vi "DrawShots_save.vi"(1 "MainCluster_IN":T11) -> (0 "MainCluster_OUT":T11)   [LabVIEW 2019]
uses:
  move_dir_ud.ctl
  73093f7f-2ca4-43a7-b6b0-9389dd3223a1.vi
  move_dir_lr.ctl
  InvaderPositionArray.ctl
  <vilib>/picture/picture.llb/imagedata.ctl
  ShotInitCluster.ctl
  CharacterCluster.ctl
  <vilib>/Utility/miscctls.llb/LVPositionTypeDef.ctl
  <vilib>/Utility/miscctls.llb/LVBoundsTypeDef.ctl
  ShotCluster.ctl
  InitCluster.ctl
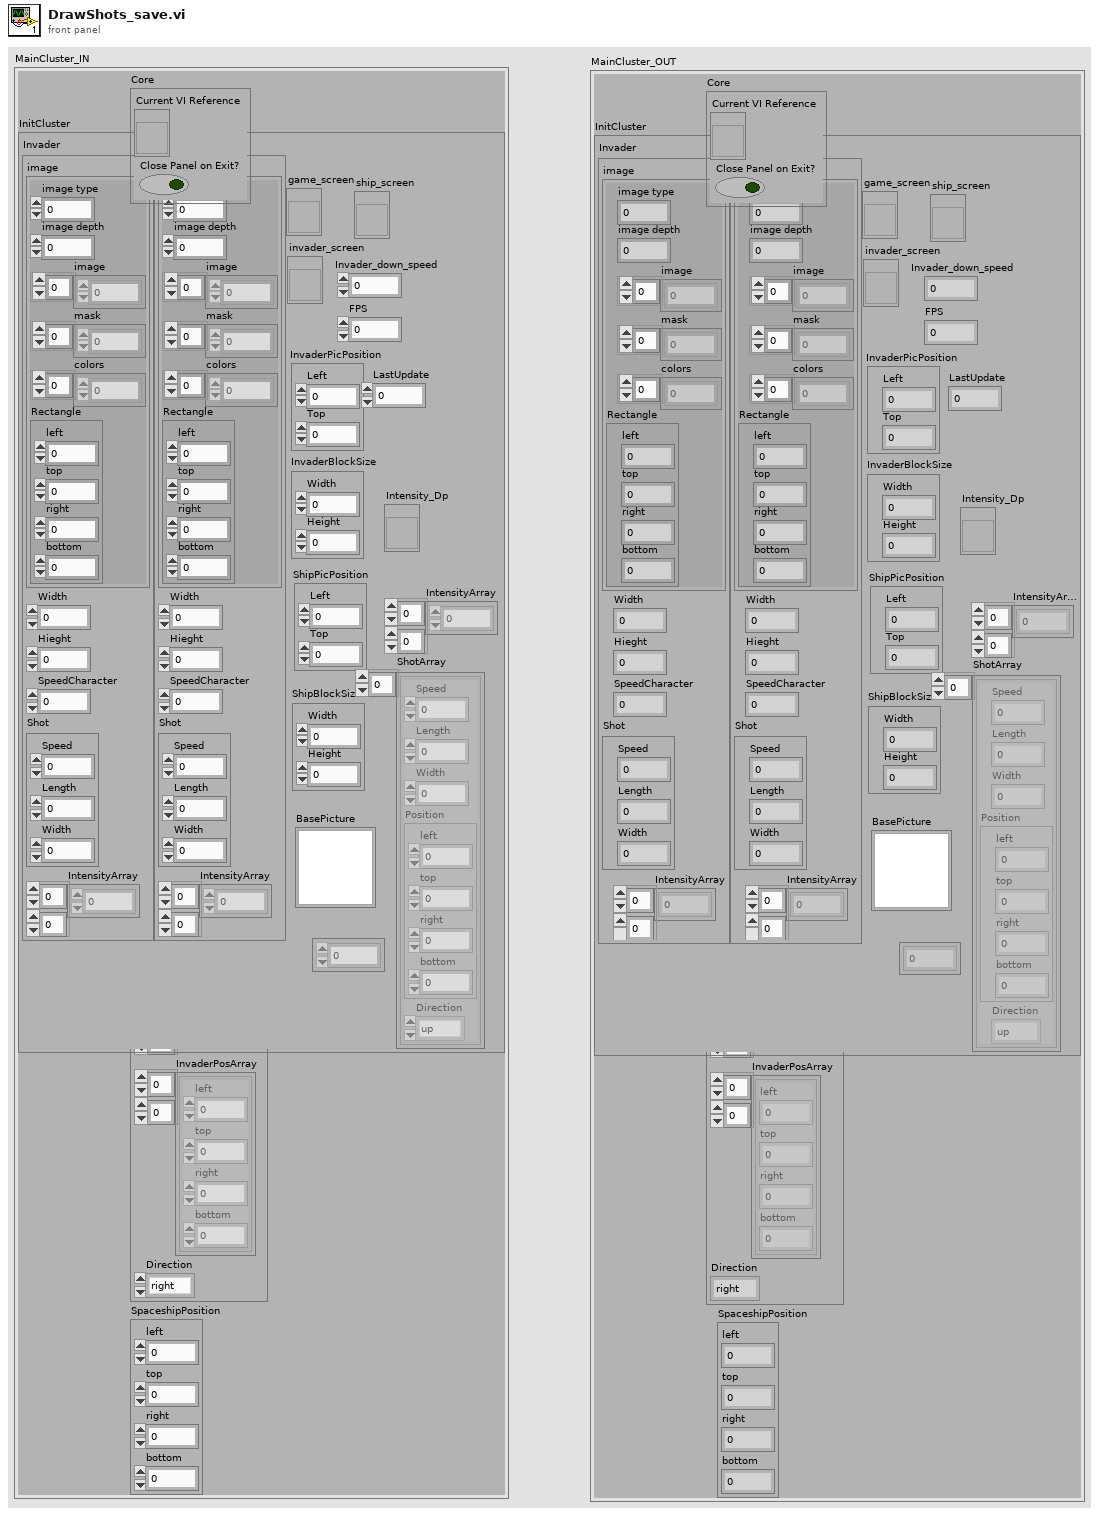
[diagram p1: front panel]
types:
  T1 = typedef "InitCluster.ctl" = cluster{"Invader":T2, "Spaceship":T2, "game_screen":refnum<vi>, "BasePicture":picture, "invader_screen":refnum<vi>, "InvaderPicPosition":T5, "Invader_down_speed":i16, "FPS":u16, "InvaderBlockSize":T6, "ship_screen":refnum<vi>, "ShipBlockSize":T6, "ShipPicPosition":T5, "LastUpdate":u32, "Intensity_Dp":refnum<vi>, "IntensityArray":u8[][], "ShotArray":T7[], "InvaderShotTimeArray":u32[]}
  T2 = typedef "CharacterCluster.ctl" = cluster{"image":T3, "Width":u32, "Hieght":u32, "SpeedCharacter":u32, "Shot":T4, "IntensityArray":u8[][]}
  T3 = typedef "imagedata.ctl" = cluster{"image type":i32, "image depth":i32, "image":u8[], "mask":u8[], "colors":u32[], "Rectangle":cluster{"left":i16, "top":i16, "right":i16, "bottom":i16}}
  T4 = typedef "ShotInitCluster.ctl" = cluster{"Speed":u32, "Length":u32, "Width":u32}
  T5 = typedef "LVPositionTypeDef.ctl" = cluster{"Left":i32, "Top":i32}
  T6 = typedef "LVBoundsTypeDef.ctl" = cluster{"Width":u32, "Height":u32}
  T7 = typedef "ShotCluster.ctl" = cluster{"Speed":u32, "Length":u32, "Width":u32, "Position":cluster{"left":i16, "top":i16, "right":i16, "bottom":i16}, "Direction":T8}
  T8 = typedef "move_dir_ud.ctl" = enum16{"up", "down"}
  T9 = typedef "InvaderPositionArray.ctl" = cluster{"InvaderAlive":bool[][], "InvaderPosArray":cluster{"left":i16, "top":i16, "right":i16, "bottom":i16}[][], "Direction":T10}
  T10 = typedef "move_dir_lr.ctl" = enum16{"right", "left"}
  T11 = cluster{"Core":cluster{"Current VI Reference":refnum<vi>, "Close Panel on Exit?":bool}, "InitCluster":T1, "InvaderPosArray":T9, "SpaceshipPosition":cluster{"left":i16, "top":i16, "right":i16, "bottom":i16}}
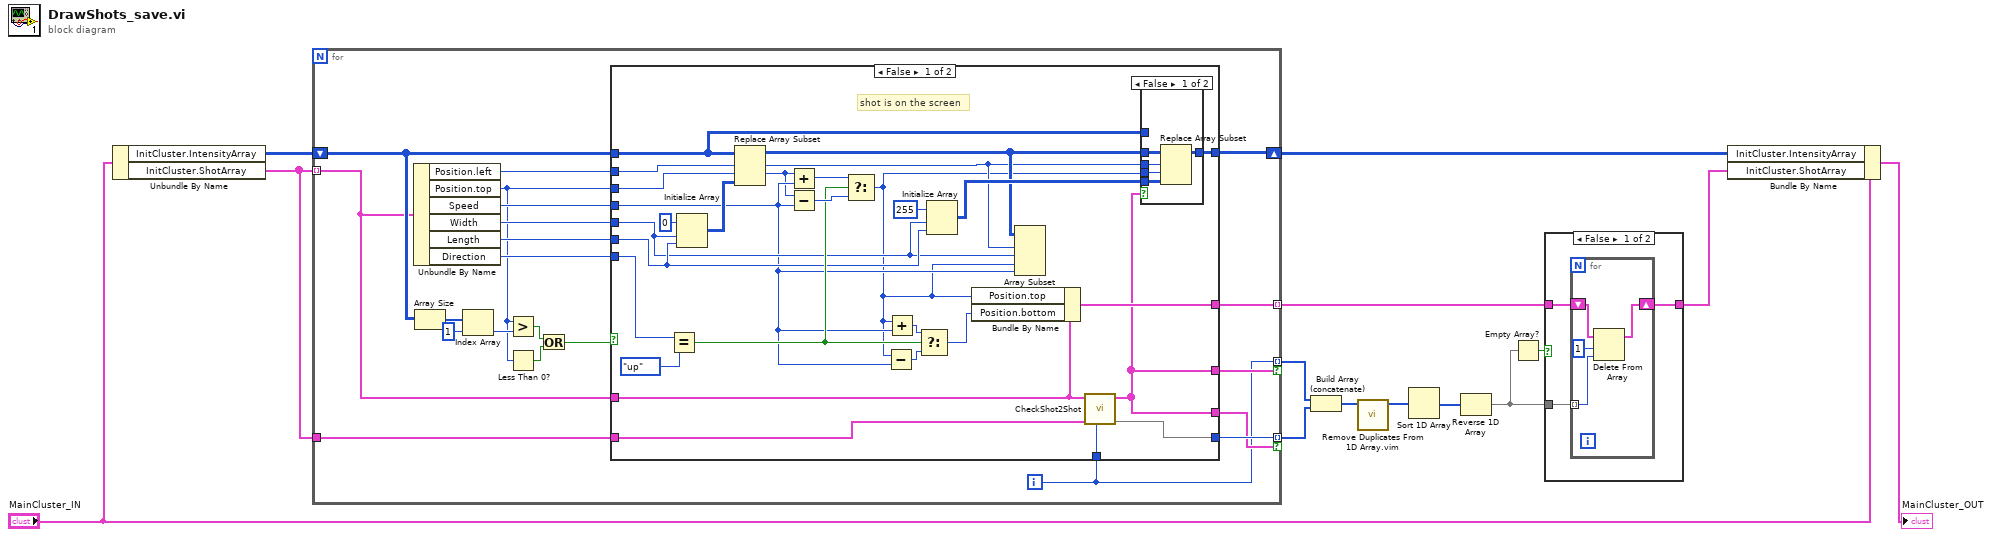
[diagram p0: block diagram]
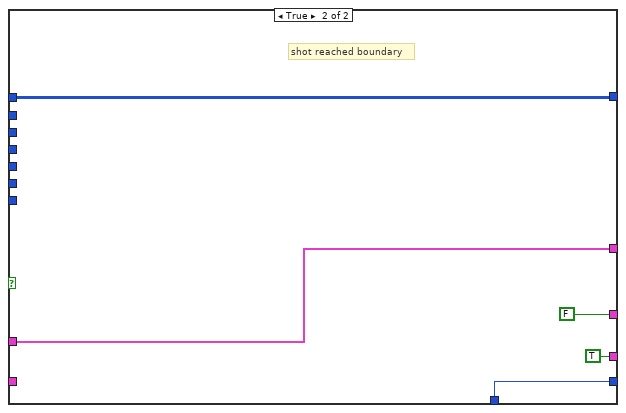
[diagram p4: hidden frame]
diagram:
  n1 = Unbundle By Name("MainCluster_IN") -> ("InitCluster.IntensityArray"=w14:u8[][], "InitCluster.ShotArray"=w10:T7[])
  n2 = for {
    tunnel: w10 -> [w18] mode=indexing
    shift-right: [w35] -> w13
    shift-left: w14 -> [w28]
    tunnel: [w33] -> w5 mode=indexing
    tunnel: w10 -> [w19]
    tunnel: [w15] -> w9 mode=indexing if=w20
    tunnel: [w17] -> w8 mode=indexing if=w16
    i -> [w15]
    n3 = Unbundle By Name(w18) -> ("Position.left"=w29:i16, "Position.top"=w24:i16, "Speed"=w30:u32, "Width"=w31:u32, "Length"=w32:u32, "Direction"=w34:T8)
    n4 = Array Size(array=w28) -> (size(s)=w27:i32[])
    n5 = Index Array(array=w27, index=1) -> (element=w25:i32)
    n6 = Greater?(x=w24, y=w25) -> (0:w23:bool)
    n7 = Less Than 0?(x=w24) -> (x < 0?=w22:bool)
    n8 = Or(x=w23, y=w22) -> (x .or. y?=w21:bool)
    n9 = case shown="False" w21 {
      tunnel: [w60 w73] -> w35
      tunnel: w34 -> [w57 _]
      tunnel: w18 -> [w37 w72]
      tunnel: [w39 w72] -> w33
      tunnel: [w38 FALSE] -> w20
      tunnel: w32 -> [w48 _]
      tunnel: w31 -> [w47 _]
      tunnel: w30 -> [w46 _]
      tunnel: w29 -> [w45 _]
      tunnel: w28 -> [w43 w73]
      tunnel: w24 -> [w44 _]
      tunnel: w19 -> [w42 _]
      tunnel: [w41 w70] -> w17
      tunnel: [w38 TRUE ("Collision")] -> w16
      tunnel: w15 -> [w40 w70]
      frame False {
        # "shot is on the screen"
        n10 = Equal?(x=w57, y=move_dir_ud."up" ("Direction")) -> (x = y?=w53:bool)
        n11 = Initialize Array(u32 0 ("element"), w47, w48) -> (w61:u32[][])
        n12 = Replace Array Subset(array=w43, new element=w61, index (row)=w45, index (col)=w44) -> (w50:u8[][])
        n13 = Add(x=w44, y=w46) -> (x+y=w55:u32)
        n14 = Subtract(x=w44, y=w46) -> (x-y=w54:u32)
        n15 = Select(t=w55, s=w53, f=w54) -> (s? t:f=w36:u32)
        n16 = Subtract(x=w36, y=w46) -> (x-y=w51:u32)
        n17 = Add(x=w36, y=w46) -> (x+y=w52:u32)
        n18 = Select(t=w52, s=w53, f=w51) -> (s? t:f=w49:u32)
        n19 = Initialize Array(u32 255 ("element"), w47, w48) -> (w58:u32[][])
        n20 = Bundle By Name(cluster=w37, "Position.top"=w36, "Position.bottom"=w49) -> (w39:T7)
        n21 = Array Subset(array=w50, index (row)=w45, length (row)=w47, index (col)=w36, length (col)=w46) -> ()  [unwired: 1 out]
        n22 = call "CheckShot2Shot.vi"(6:w40, 8:w42, "ShotArray_IN"=w37) -> (0:w41, "ShotArray_OUT"=w38:T7[])  [unwired: 7 in]
        n23 = case shown="False" w38 {
          tunnel: [w67 w68] -> w60
          tunnel: w58 -> [w66 _]
          tunnel: w50 -> [w65 w68]
          tunnel: w45 -> [w64 _]
          tunnel: w36 -> [w63 _]
          tunnel: w43 -> [_ _]
          frame False {
            n24 = Replace Array Subset(array=w65, new element=w66, index (row)=w64, index (col)=w63) -> (w67:u8[][])
          }
          frame True {
          }
        }
      }
      frame True {
        # "shot reached boundary"
      }
    }
  }
  n25 = Build Array (concatenate)(w9, w8) -> (w3:i32[])
  n26 = call "Remove Duplicates From 1D Array.vim"("array"=w3) -> ("array with duplicates removed"=w7:i32[])  [unwired: 10 in]
  n27 = Sort 1D Array(array=w7) -> (sorted array=w6:i32[])
  n28 = Reverse 1D Array(array=w6) -> (reversed array=w2:i32[])
  n29 = Empty Array?(array=w2) -> (empty?=w1:bool)
  n30 = case shown="False" w1 {
    tunnel: w2 -> [w76 _]
    tunnel: w5 -> [w75 w81]
    tunnel: [w74 w81] -> w4
    frame False {
      n31 = for {
        tunnel: w76 -> [w79] mode=indexing
        shift-right: [w77] -> w74
        shift-left: w75 -> [w80]
        n32 = Delete From Array(array=w80, length=1, index=w79) -> (array with subset deleted=w77:T7[])  [unwired: 1 out]
      }
    }
    frame True {
    }
  }
  n33 = Bundle By Name(cluster="MainCluster_IN", "InitCluster.IntensityArray"=w13, "InitCluster.ShotArray"=w4) -> (→"MainCluster_OUT":T11)
